vi "omega_sub_Encoder_4096ppr.vi"(5 "mt0":u32, 7 "omega_pre":fxp<+/-,20,9>, 8 "ticks_m_pre":u32, 9 "ticks":u32, 10 "count_pre":i32, 11 "count":i32) -> (0 "ticks_m":u32, 1 "mt":u32, 3 "omega":fxp<+/-,20,9>)   [LabVIEW 2014]
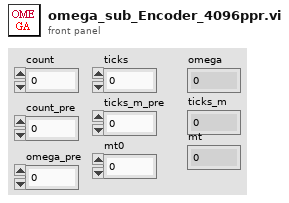
[diagram p1: front panel]
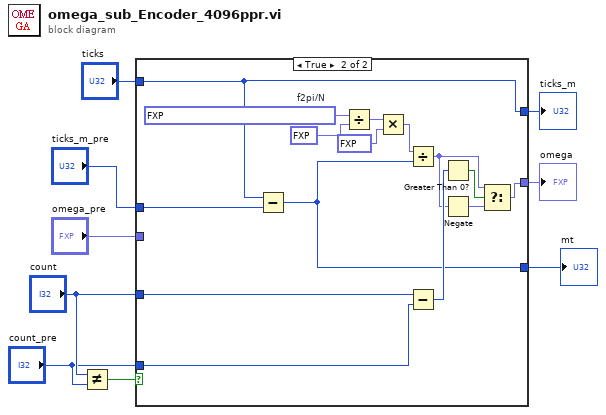
[diagram p0: block diagram]
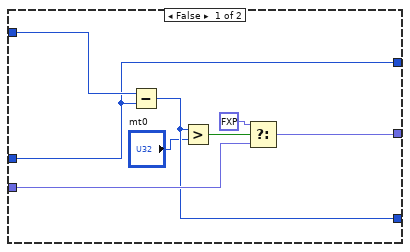
[diagram p2: hidden frame]
diagram:
  n1 = Not Equal?(x="count", y="count_pre") -> (x != y?=w9:bool)
  n2 = case shown="True" w9 {
    tunnel: "ticks" -> [w17 w29]
    tunnel: "count" -> [_ w32]
    tunnel: "count_pre" -> [_ w31]
    tunnel: [w16 w29] -> w2
    tunnel: "ticks_m_pre" -> [w16 w28]
    tunnel: [w13 w24] -> w6
    tunnel: "omega_pre" -> [w14 _]
    tunnel: [w11 w23] -> w1
    frame False {
      n3 = Subtract(x=w17, y=w16) -> (x-y=w11:u32)
      n4 = Greater?(x=w11, y="mt0") -> (0:w15:bool)
      n5 = Select(t=fxp<+/-,20,9> 0.0, s=w15, f=w14) -> (s? t:f=w13:fxp<+/-,20,9>)
    }
    frame True {
      w22 = fxp<+,40,19> 314159.26535892487  # f2pi/N
      n6 = Subtract(x=w29, y=w28) -> (x-y=w23:u32)
      n7 = Divide(x=w22, y=fxp<+,40,19> 800.0) -> (x/y=w20:fxp<+,64,40>)
      n8 = Multiply(x=w20, y=fxp<+,64,40> 4096.0) -> (x*y=w18:fxp<+,64,80>)
      n9 = Divide(x=w18, y=w23) -> (x/y=w26:fxp<+/-,20,9>)
      n10 = Subtract(x=w32, y=w31) -> (x-y=w30:i32)
      n11 = Greater Than 0?(x=w30) -> (x > 0?=w25:bool)
      n12 = Negate(x=w26) -> (-x=w27:fxp<+/-,20,9>)
      n13 = Select(t=w26, s=w25, f=w27) -> (s? t:f=w24:fxp<+/-,20,9>)
    }
  }
  "omega" <- w6
  "ticks_m" <- w2
  "mt" <- w1
